vi "Apply Constants.vi"(2 "Module Number":i32, 3 "constants cluster":cluster{"a":dbl, "b":dbl, "c":dbl, "d":dbl}, 4 "Max Speed or 1":dbl) -> (0 "Magnitude":dbl format="%#_13g", 1 "Desired Direction (rad)":dbl format="%#_13g")   [LabVIEW 2016]
uses:
  <vilib>/ptbypt/NI_PtbyPt.lvlib
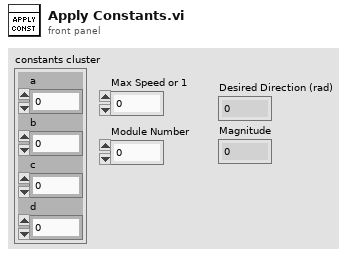
[diagram p1: front panel]
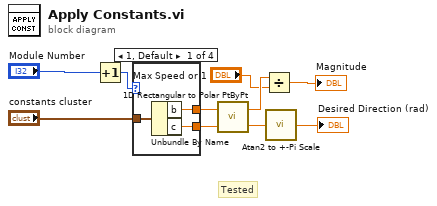
[diagram p0: block diagram]
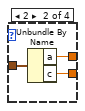
[diagram p2: hidden frame]
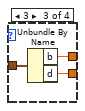
[diagram p3: hidden frame]
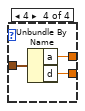
[diagram p4: hidden frame]
diagram:
  # "Tested"
  n1 = Increment(x="Module Number") -> (x+1=w9:i32)
  n2 = case shown="1, Default" w9 {
    tunnel: "constants cluster" -> [w13 w16 w19 w22]
    tunnel: [w12 w15 w18 w21] -> w7
    tunnel: [w11 w14 w17 w20] -> w6
    frame 1, Default {
      n3 = Unbundle By Name(w13) -> ("b"=w12:dbl, "c"=w11:dbl)
    }
    frame 2 {
      n4 = Unbundle By Name(w16) -> ("a"=w15:dbl, "c"=w14:dbl)
    }
    frame 3 {
      n5 = Unbundle By Name(w19) -> ("b"=w18:dbl, "d"=w17:dbl)
    }
    frame 4 {
      n6 = Unbundle By Name(w22) -> ("a"=w21:dbl, "d"=w20:dbl)
    }
  }
  n7 = call <vilib>:"1D Rectangular to Polar PtByPt.vi"("y"=w6, "x"=w7) -> ("phase"=w3:dbl, "magnitude"=w5:dbl)
  n8 = Divide(x=w5, y="Max Speed or 1") -> (x/y=→"Magnitude":dbl)
  n9 = call "Atan2 to +-Pi Scale.vi"("atan2 result"=w3) -> ("Scaled"=→"Desired Direction (rad)":dbl)
